vi "Tree add tags.vi"(8 "error in (no error)":errorcluster, 9 "Table":cluster{"Table":string, "alias":string}[](array[cluster]), 10 "Line_Name":string, 11 "specific class reference":refnum<vi>) -> (0 "error out":errorcluster, 3 "Tree out":refnum<vi>)   [LabVIEW 2014]
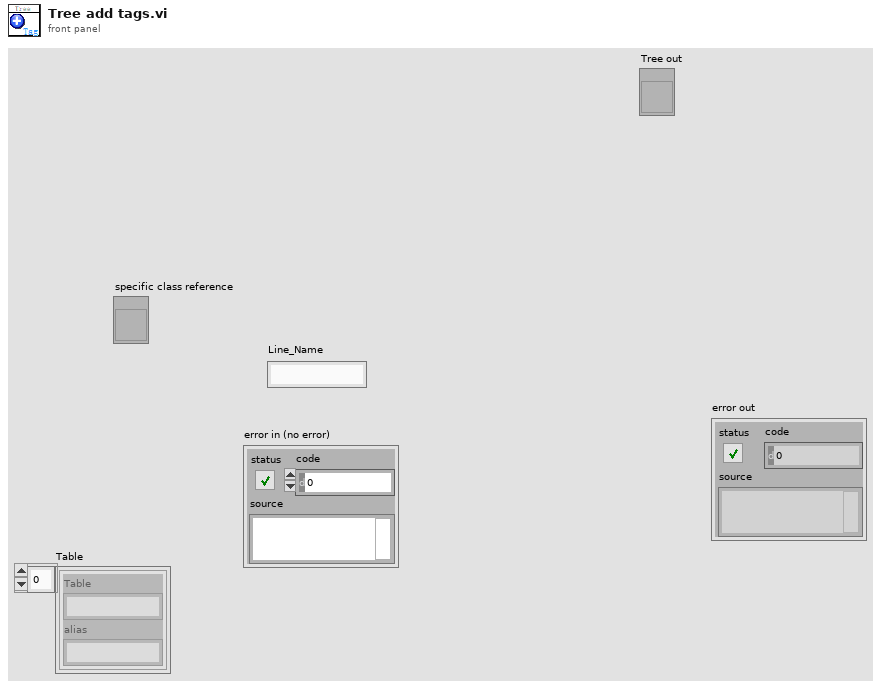
[diagram p1: front panel]
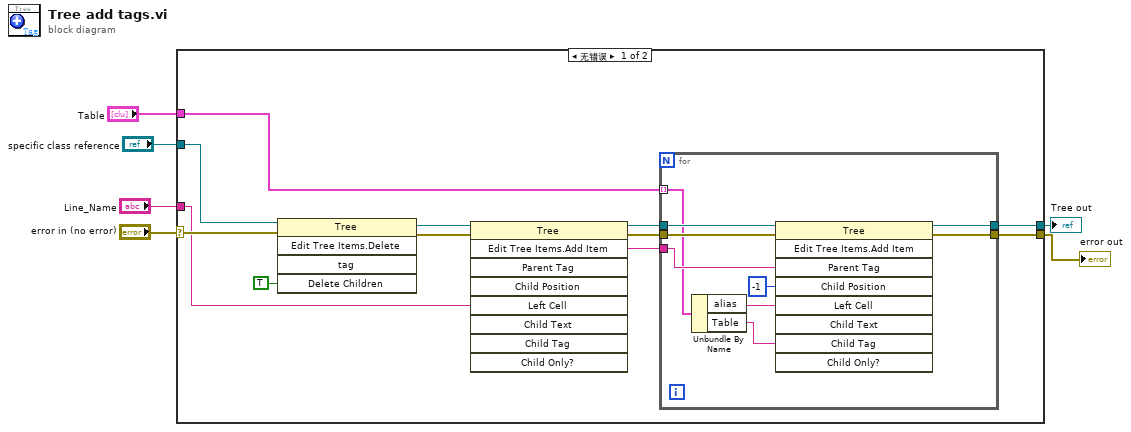
[diagram p0: block diagram]
diagram:
  n1 = case shown="无错误" "error in (no error)" {
    selector: "error in (no error)" -> [w18 w28]
    tunnel: "specific class reference" -> [w17 w29]
    tunnel: "Line_Name" -> [w13 _]
    tunnel: "Table" -> [w7 _]
    tunnel: [w9 w29] -> w2
    tunnel: [w8 w28] -> w1
    frame No Error {
      n2 = invoke class="Tree" method="Edit Tree Items.Delete"(reference=w17, error in=w18, "Delete Children"=TRUE ("Delete Children?")) -> (reference out=w14:refnum<vi>, error out=w15:errorcluster)  [unwired: 2 in, 3 out]
      n3 = invoke class="Tree" method="Edit Tree Items.Add Item"(reference=w14, error in=w15, "Left Cell"=w13) -> (reference out=w11:refnum<vi>, error out=w12:errorcluster, "Edit Tree Items:Add Item"=w10:string)  [unwired: 6 in, 6 out]
      n4 = for {
        tunnel: w7 -> [w24] mode=indexing
        tunnel: w12 -> [w27]
        tunnel: w11 -> [w26]
        tunnel: w10 -> [w25]
        tunnel: [w20] -> w8
        tunnel: [w19] -> w9
        n5 = Unbundle By Name(w24) -> ("alias"=w23:string, "Table"=w22:string)
        n6 = invoke class="Tree" method="Edit Tree Items.Add Item"(reference=w26, error in=w27, "Parent Tag"=w25, "Child Position"=-1, "Left Cell"=w23, "Child Tag"=w22) -> (reference out=w19:refnum<vi>, error out=w20:errorcluster)  [unwired: 3 in, 7 out]
      }
    }
    frame Error {
    }
  }
  "error out" <- w1
  "Tree out" <- w2
